vi "Process.vi"(2 "acq":refnum<class "niUSRP Rx DSP v2 FPGA.lvclass">) -> ()   [LabVIEW 2025, in "niUSRP Rx DSP v2 FPGA.lvclass"]
uses:
  niUSRP Rx DSP v2 FPGA.lvclass
  <instrlib>/_niInstr/Basic Elements/v1/FPGA/niInstr Basic Elements v1 FPGA.lvlib
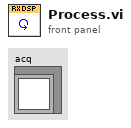
[diagram p1: front panel]
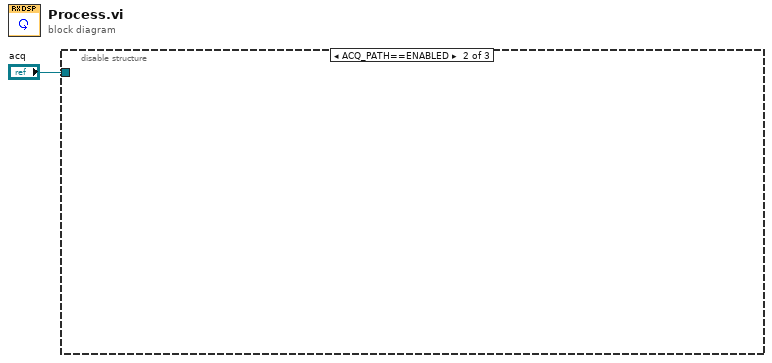
[diagram p0: block diagram]
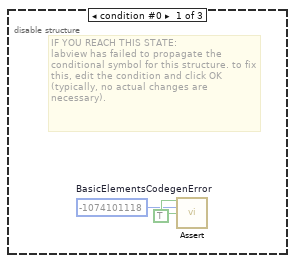
[diagram p2: hidden frame]
diagram:
  n1 = disable-structure shown="ACQ_PATH==ENABLED" {
    disable-tunnel: "acq" -> [_ _ _]
    frame condition #0 {
      w3 = TRUE ("assert")
      w2 = -1074101118  # BasicElementsCodegenError
      # "IF YOU REACH THIS STATE:\nlabview has failed to propagate the conditional symbol for this structure. to fix this, edit the condition and click OK (typically, no actual changes are necessary)."
      n2 = call <instrlib>:"Assert.vi"("assert"=w3, "error code"=w2, "enable show error"=w3) -> ()  [unwired: 13 in]
    }
    frame condition #1 (active) {
    }
    frame condition #2 {
    }
  }
